vi "Rio_Trapazodial_Velocity.vi"() -> ()   [LabVIEW 2017]
uses:
  <vilib>/Analysis/1siggen.llb/Ramp Pattern by Samples.vi
  <vilib>/Analysis/NI_AALBase.lvlib
panel:
  in  "Constant":dbl
  out "Waveform Graph":dbl[](graph)
  in  "Max V":dbl
  in  "End":dbl
  in  "Start":dbl
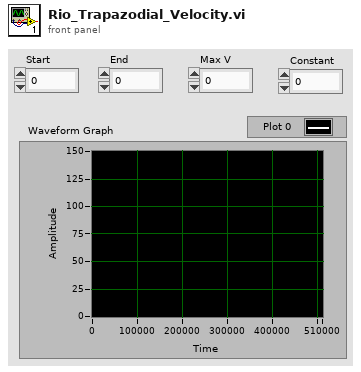
[diagram p1: front panel]
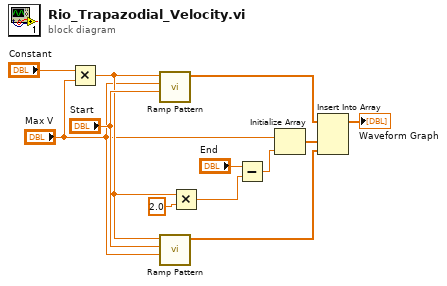
[diagram p0: block diagram]
diagram:
  n1 = Multiply(x="Constant", y="Max V") -> (x*y=w3:dbl)
  n2 = call-poly <vilib>:"Ramp Pattern.vi"("start"="Start", "end"="Max V", "samples"=w3) -> ("Ramp Pattern"=w11:dbl[])  [unwired: 7 in, 1 out]
  n3 = call-poly <vilib>:"Ramp Pattern.vi"("start"="Max V", "end"="Start", "samples"=w3) -> ("Ramp Pattern"=w9:dbl[])  [unwired: 7 in, 1 out]
  n4 = Multiply(x=w3, y=2.0) -> (x*y=w5:dbl)
  n5 = Subtract(x="End", y=w5) -> (x-y=w6:dbl)
  n6 = Initialize Array("Max V", w6) -> (w10:dbl[])
  n7 = Insert Into Array(array=w11, new element #1=w10, new element #2=w9) -> (→"Waveform Graph":dbl[])  [unwired: 1 in]
